vi "p30 posicion araña.vi"() -> ()   [LabVIEW 2013]
uses:
  <vilib>/Math Plots/3D Math Plots/3D Mesh/3D Mesh Datatype/3D Mesh Datatype.lvclass
  <vilib>/Math Plots/3D Math Plots/3D Mesh/3D Mesh Datatype/Public/Plot Helper (Matrix).vi
  <vilib>/Math Plots/3D Math Plots/3D Mesh/3D Mesh XCtrl/3D Mesh.xctl
panel:
  out "sum":u32
  out "Array 4":dbl[](array[numeric])
  out "appended path":path
  out "Array 2":dbl[](array[numeric])
  out "Array":dbl[](array[numeric])
  out "XY Graph":cluster{dbl[], dbl[]}(graph)
  in  "path to BMP file 3":path
  out "Waveform Chart 2":dbl[](graph)
  out "Waveform Chart":dbl[](graph)
  out "3D Mesh":refnum<class "3D Plot Datatype.lvclass">[](xcontrol)
  in  "Slide":dbl(slide) scale=0.0..255.0
  out "new picture":picture
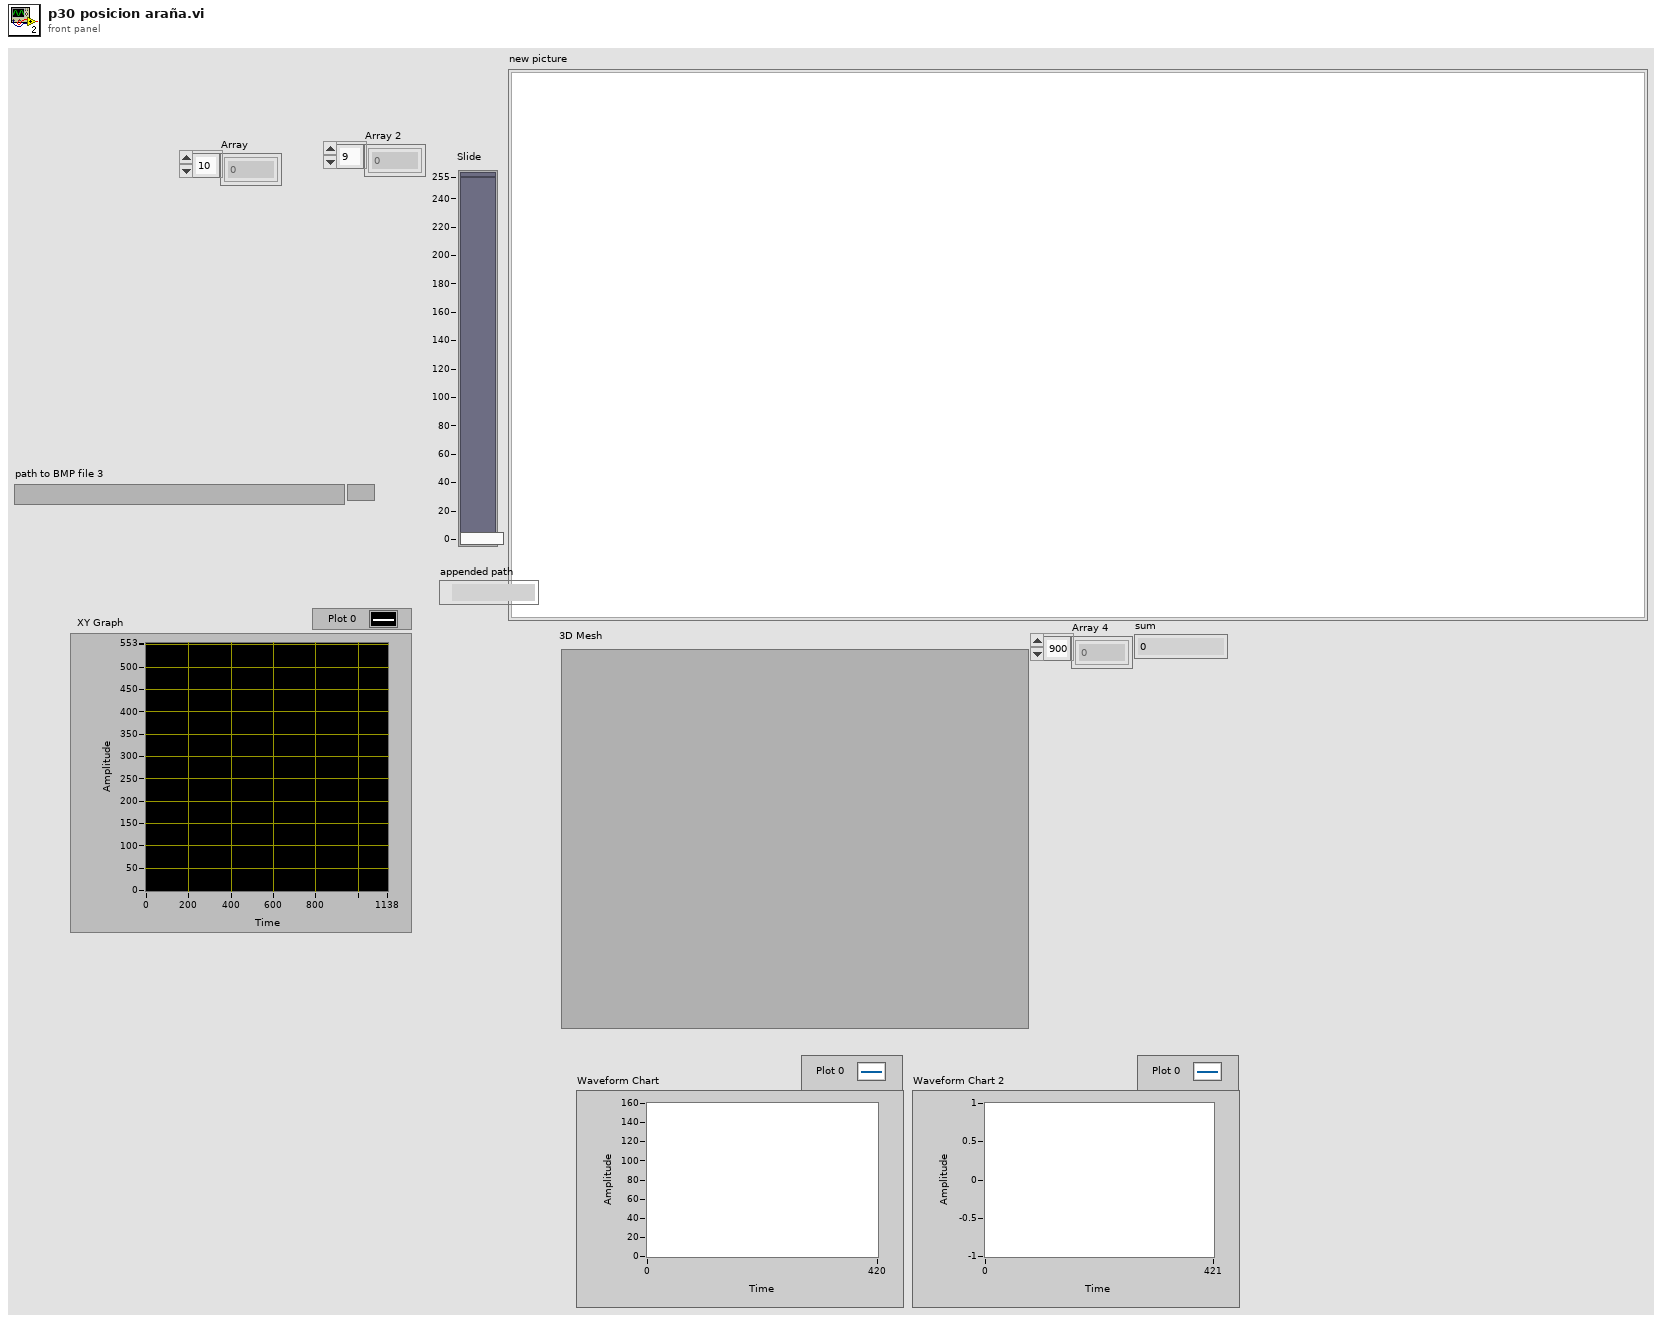
[diagram p1: front panel]
types:
  T1 = typedef "imagedata.ctl" = cluster{"image type":i32, "image depth":i32, "image":u8[], "mask":u8[], "colors":u32[], "Rectangle":cluster{"left":i16, "top":i16, "right":i16, "bottom":i16}}
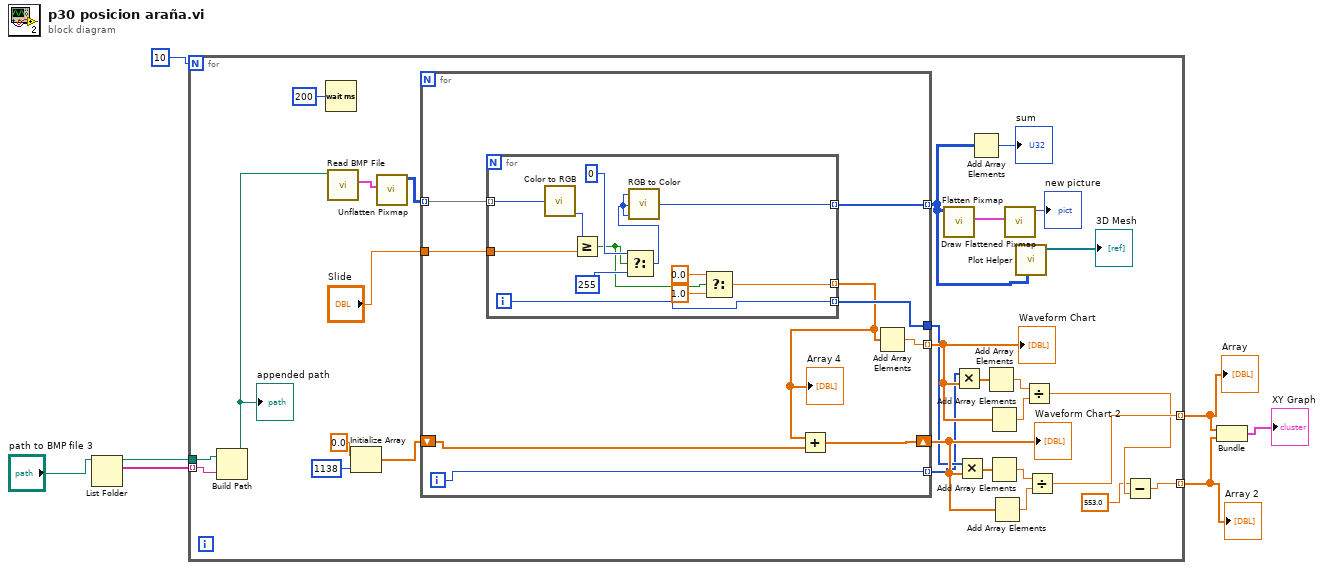
[diagram p0: block diagram]
diagram:
  n1 = List Folder(path="path to BMP file 3") -> (path out=w6:path, filenames=w4:string[])  [unwired: 3 in, 2 out]
  n2 = for {
    N: 10 -> [_]
    tunnel: w6 -> [w31]
    tunnel: w4 -> [w30] mode=indexing
    tunnel: [w11] -> w3 mode=indexing
    tunnel: [w10] -> w2 mode=indexing
    n3 = Build Path(base path=w31, name or relative path=w30) -> (appended path=w29:path)
    "appended path" <- w29
    n4 = Wait (ms)(milliseconds to wait=u32 200) -> ()  [unwired: 1 out]
    n5 = call <vilib>:"Read BMP File.vi"("path to BMP file"=w29) -> ("image data"=w32:T1)  [unwired: 8 in, 2 out]
    n6 = Initialize Array(0.0 ("element"), 1138 ("dimension size")) -> (w16:dbl[])
    n7 = call <vilib>:"Unflatten Pixmap.vi"("image data"=w32) -> ("24-bit pixmap"=w28:u32[][])  [unwired: 4 in, 6 out]
    n8 = for {
      tunnel: w28 -> [w45] mode=indexing
      tunnel: [w42] -> w15 mode=indexing
      tunnel: "Slide" -> [w44]
      tunnel: [w43] -> w26 mode=indexing
      shift-right: [w40] -> w19
      shift-left: w16 -> [w41]
      tunnel: [w39] -> w13
      tunnel: [w38] -> w12 mode=indexing
      i -> [w38]
      n9 = for {
        tunnel: w45 -> [w57] mode=indexing
        tunnel: [w53] -> w42 mode=indexing
        tunnel: w44 -> [w56]
        tunnel: [w47] -> w37 mode=indexing
        tunnel: [w46] -> w39 mode=indexing
        i -> [w46]
        n10 = call <vilib>:"Color to RGB.vi"("Color"=w57) -> ("B"=w54:u8)  [unwired: 3 out]
        n11 = Greater Or Equal?(x=w54, y=w56) -> (x >= y?=w50:bool)
        n12 = Select(t=0, s=w50, f=255) -> (s? t:f=w51:i32)
        n13 = call <vilib>:"RGB to Color.vi"("B"=w51, "G"=w51, "R"=w51) -> ("Color"=w53:u32)
        n14 = Select(t=0.0, s=w50, f=1.0) -> (s? t:f=w47:dbl)
      }
      "Array 4" <- w37
      n15 = Add(x=w37, y=w41) -> (x+y=w40:dbl[])
      n16 = Add Array Elements(numeric array=w37) -> (sum=w43:dbl)
    }
    "Waveform Chart" <- w26
    "Waveform Chart 2" <- w19
    n17 = call <vilib>:"Flatten Pixmap.vi"("24-bit pixmap"=w15) -> ("image data"=w36:T1)  [unwired: 10 in]
    n18 = Multiply(x=w12, y=w26) -> (x*y=w27:dbl[])
    n19 = Multiply(x=w13, y=w19) -> (x*y=w21:dbl[])
    n20 = Add Array Elements(numeric array=w15) -> (sum=→"sum":u32)
    n21 = Add Array Elements(numeric array=w27) -> (sum=w25:dbl)
    n22 = Add Array Elements(numeric array=w26) -> (sum=w24:dbl)
    n23 = Add Array Elements(numeric array=w21) -> (sum=w22:dbl)
    n24 = Add Array Elements(numeric array=w19) -> (sum=w23:dbl)
    n25 = call <vilib>:"Draw Flattened Pixmap.vi"("image data"=w36) -> ("new picture"=→"new picture":picture)  [unwired: 8 in]
    n26 = call-poly <vilib>:"Plot Helper.vi"("z matrix"=w15) -> ("3D Plot lvclass Array out"=→"3D Mesh":refnum<class "3D Plot Datatype.lvclass">[])  [unwired: 5 in, 5 out]
    n27 = Divide(x=w25, y=w24) -> (x/y=w9:dbl)
    n28 = Divide(x=w22, y=w23) -> (x/y=w11:dbl)
    n29 = Subtract(x=553.0 ("y"), y=w9) -> (x-y=w10:dbl)
  }
  "Array" <- w3
  "Array 2" <- w2
  n30 = Bundle(w3, w2) -> (→"XY Graph":cluster{dbl[], dbl[]})  [unwired: 1 in]
